vi "jsonParseU64.vi"(8 "error in (no error)":errorcluster, 10 "path":string, 11 "d in":i64) -> (0 "error out":errorcluster, 1 "found?":bool, 2 "value":u64, 3 "d out":i64)   [LabVIEW 2015, in "rapidjson wrapper.lvlib"]
uses:
  rapidjson wrapper.lvlib
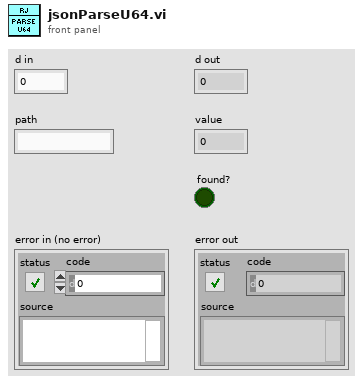
[diagram p1: front panel]
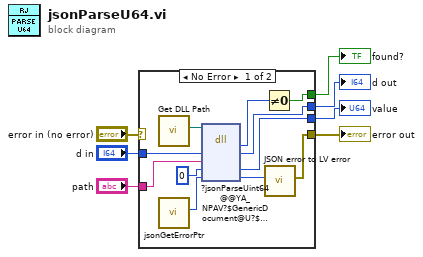
[diagram p0: block diagram]
diagram:
  n1 = case shown="No Error" "error in (no error)" {
    selector: "error in (no error)" -> [_ w20]
    tunnel: [w16 w20] -> w6
    tunnel: [w8 _] -> w3
    tunnel: "d in" -> [w14 w19]
    tunnel: "path" -> [w13 _]
    tunnel: [w12 w19] -> w4
    tunnel: [w11 _] -> w5
    frame No Error {
      n2 = call "Get DLL Path.vi"() -> ("Path"=w18:path)  [unwired: 11 in]
      n3 = call "jsonGetErrorPtr.vi"() -> ("return type"=w15:i64)  [unwired: 10 in, 1 out]
      n4 = dll-call lib="C:/Users/tblair/Documents/Git Projects/rapidjson-for-LabVIEW/lvrjs/Debug/lvrjs.dll" fn="?jsonParseUint64@@YA_NPAV?$GenericDocument@U?$UTF8@D@rapidjson@@V?$MemoryPoolAllocator@VCrtAllocator@rapidjson@@@2@VCrtAllocator@2@@rapidjson@@PADAA_K0@Z"(path in=w18, "d"=w14, "path"=w13, "value"=u64 0, "error"=w15) -> ("return type"=w10:i32, "d"=w12:i64, "value"=w8:u64, "error"=w17:i64)  [unwired: 3 in, 2 out]
      n5 = Not Equal To 0?(x=w10) -> (x != 0?=w11:bool)
      n6 = call "JSON error to LV error.vi"("jsonError"=w17) -> ("error out"=w16:errorcluster)  [unwired: 10 in]
    }
    frame Error {
    }
  }
  "error out" <- w6
  "value" <- w3
  "d out" <- w4
  "found?" <- w5
